vi "Laplacian Example.vi"() -> ()   [LabVIEW 2012]
uses:
  User Controls/Array Dimensions.ctl
  Non-User VIs/Allocate Memory/AllocateMemory_32f.vi
  Non-User VIs/Functions/Laplacian/Create Laplacian 32f.vi
  Non-User VIs/Functions/Laplacian/Delete Laplacian 32f.vi
  Non-User VIs/Error Checking/View Error Log Mode Functional Global.vi
  Non-User VIs/Write Memory/WriteMemory_32f.vi
  Non-User VIs/Functions/Laplacian/Compute Laplacian 32f.vi
  Non-User VIs/Read Memory/ReadMemory_32f.vi
  OpenCLV x64.lvlib
panel:
  out "Laplacian":sgl[][][](array[numeric])
  out "Time in ms":u32=149
  in  "Dimension":T1={"Depth"=97, "Height"=512, "Width"=191} {"Width" min=1; "Height" min=1; "Depth" min=1}
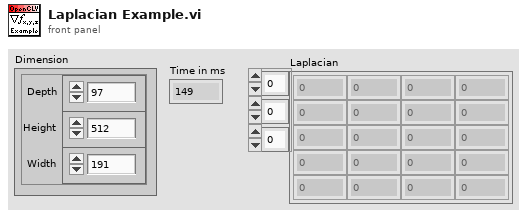
[diagram p1: front panel]
types:
  T1 = typedef "Array Dimensions.ctl" = cluster{"Depth":u64, "Height":u64, "Width":u64}
  T2 = typedef "OpenCLV x64.lvlib/Device ID.ctl" = u64
  T3 = typedef "OpenCLV x64.lvlib/Memory Object.ctl" = cluster{"Device ID":T2, "Memeroy ID":T4, "Dimension":T1, "Memory Type":T5}
  T4 = typedef "OpenCLV x64.lvlib/Memory ID.ctl" = u64
  T5 = typedef "OpenCLV x64.lvlib/Memory Type.ctl" = enum16{"32f", "u8", "i8", "u16", "i16", "u32", "i32", "64f"}
  T6 = typedef "OpenCLV x64.lvlib/Laplacian Object.ctl" = cluster{"Device Out":T2, "Program Handle":T7, "Laplacian Out":T3}
  T7 = typedef "OpenCLV x64.lvlib/Program Handle.ctl" = u64
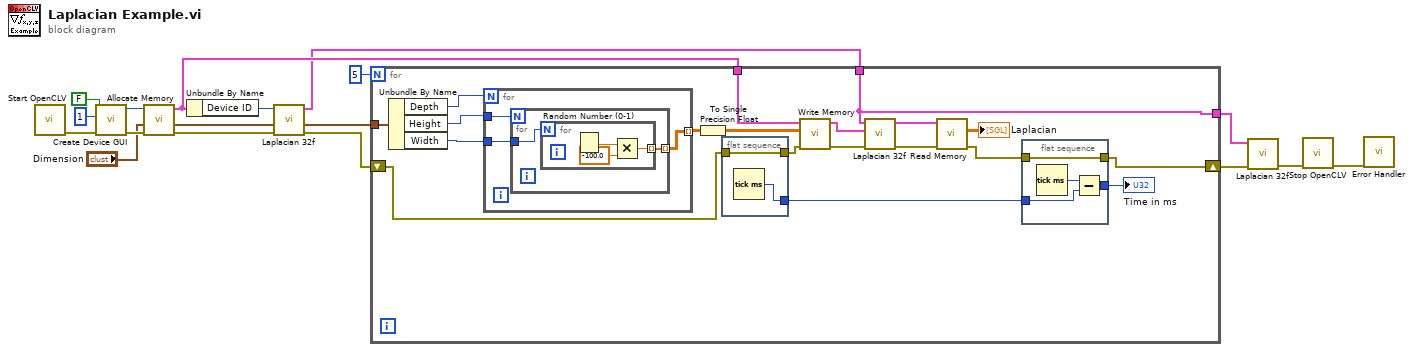
[diagram p0: block diagram]
diagram:
  n1 = call "Start OpenCLV.vi"() -> ("Error Out"=w18:errorcluster)  [unwired: 11 in]
  n2 = call "Create Device GUI.vi"("Error In"=w18, "Platform"=1, "Skip Configuration"=FALSE) -> ("error constant"=w17:errorcluster, "Device Reference"=w16:T2)  [unwired: 7 in]
  n3 = call-poly "Allocate Memory.vi"("Error In"=w17, "Dimension"="Dimension", "Device In"=w16) -> ("Error Out"=w11:errorcluster, "Dimension Out"=w9:T1, "Memory Object"=w8:T3)  [unwired: 6 in]
  n4 = Unbundle By Name(w8) -> ("Device ID"=w6:T2)
  n5 = call-poly "Laplacian 32f.vi"("Error In"=w11, "Dimension"=w9, "Device In"=w6) -> ("Error Out"=w10:errorcluster, "Dimension Out"=w3:T1, "Laplacian Out"=w5:T6)  [unwired: 6 in]
  n6 = for {
    N: 5 -> [_]
    tunnel: [w34] -> w4
    tunnel: w5 -> [w34]
    tunnel: w3 -> [w32]
    tunnel: w8 -> [w31]
    shift-right: [w19] -> w2
    shift-left: w10 -> [w23]
    n7 = Unbundle By Name(w32) -> ("Depth"=w37:u64, "Height"=w36:u64, "Width"=w35:u64)
    n8 = for {
      N: w37 -> [_]
      tunnel: w36 -> [w46]
      tunnel: w35 -> [w45]
      tunnel: [w44] -> w33 mode=indexing
      n9 = for {
        N: w46 -> [_]
        tunnel: w45 -> [w48]
        tunnel: [w47] -> w44 mode=indexing
        n10 = for {
          N: w48 -> [_]
          tunnel: [w49] -> w47 mode=indexing
          n11 = Random Number (0-1)() -> (number: 0 to 1=w51:dbl)
          n12 = Multiply(x=w51, y=-100.0) -> (x*y=w49:dbl)
        }
      }
    }
    n13 = To Single Precision Float(number=w33) -> (single precision float=w30:sgl[][][])
    n14 = flat-sequence {
      tunnel: [w43] -> w24
      tunnel: w23 -> [w43]
      tunnel: [w42] -> w21
      frame #0 {
        n15 = Tick Count (ms)() -> (millisecond timer value=w42:u32)
      }
    }
    n16 = call-poly "Write Memory.vi"("Error In"=w24, "Data In"=w30, "Memory Object In"=w31) -> ("Error Out"=w26:errorcluster, "Memory Object Out"=w25:T3)  [unwired: 6 in, 1 out]
    n17 = call-poly "Laplacian 32f.vi"("Error In"=w26, "Input"=w25, "Laplacian Object"=w34) -> ("Error Out"=w29:errorcluster, "Laplacian Out"=w28:T3)  [unwired: 6 in, 1 out]
    n18 = call-poly "Read Memory.vi"("Error In"=w29, "Memory Object In"=w28) -> ("Error Out"=w22:errorcluster, "Data Out"=→"Laplacian":sgl[][][])  [unwired: 6 in, 2 out]
    n19 = flat-sequence {
      tunnel: w22 -> [w38]
      tunnel: w21 -> [w40]
      tunnel: [w39] -> w20
      tunnel: [w38] -> w19
      frame #0 {
        n20 = Tick Count (ms)() -> (millisecond timer value=w41:u32)
        n21 = Subtract(x=w41, y=w40) -> (x-y=w39:u32)
      }
    }
    "Time in ms" <- w20
  }
  n22 = call-poly "Laplacian 32f.vi"("Error In"=w2, "Laplacian Object"=w4) -> ("Error Out"=w14:errorcluster)  [unwired: 9 in]
  n23 = call "Stop OpenCLV.vi"("Error In"=w14) -> ("Error Out"=w1:errorcluster)  [unwired: 10 in]
  n24 = call-poly "Error Handler.vi"("Error In"=w1) -> ()  [unwired: 10 in, 1 out]
